vi "turret limit.vi"(2 "limit":dbl, 3 "output speed":dbl, 4 "Current Rate in":dbl, 5 "Distance":dbl) -> (0 "limited output speed":dbl, 1 "Current Rate out":dbl)   [LabVIEW 2011]
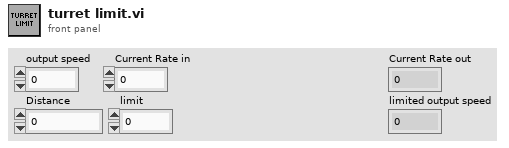
[diagram p1: front panel]
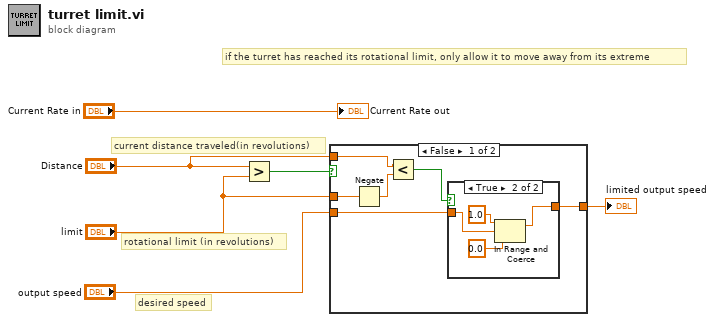
[diagram p0: block diagram]
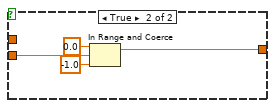
[diagram p3: hidden frame]
diagram:
  # "desired speed"
  # "rotational limit (in revolutions)"
  # "current distance traveled(in revolutions)"
  # "if the turret has reached its rotational limit, only allow it to move away from its extreme"
  n1 = Greater?(x="Distance", y="limit") -> (0:w5:bool)
  n2 = case shown="False" w5 {
    tunnel: "output speed" -> [w8 w21]
    tunnel: "Distance" -> [w12 _]
    tunnel: "limit" -> [w11 _]
    tunnel: [w7 w18] -> w1
    frame False {
      n3 = Negate(x=w11) -> (-x=w9:dbl)
      n4 = Less?(x=w12, y=w9) -> (x < y?=w10:bool)
      n5 = case shown="True" w10 {
        tunnel: w8 -> [w13 w15]
        tunnel: [w13 w14] -> w7
        frame False {
        }
        frame True {
          n6 = In Range and Coerce(upper limit=1.0, x=w15, lower limit=0.0) -> (coerced(x)=w14:dbl)  [unwired: 1 out]
        }
      }
    }
    frame True {
      n7 = In Range and Coerce(upper limit=0.0, x=w21, lower limit=-1.0) -> (coerced(x)=w18:dbl)  [unwired: 1 out]
    }
  }
  "limited output speed" <- w1
  "Current Rate out" <- "Current Rate in"
